vi "Update Configuration.vi"(8 "error in (no error)":errorcluster, 10 "FP Configuration":T1, 11 "Control In":refnum<class "Control.lvclass">) -> (0 "error out":errorcluster, 3 "Control In":refnum<class "Control.lvclass">)   [LabVIEW 2015, in "Front Panel Publisher.lvlib" / "Control.lvclass"]
uses:
  Control.lvclass
  Web Front Panel_class/Controls/FP Object Configuration.ctl
  Object_class/Object.lvclass
  Front Panel Publisher.lvlib
  Web Front Panel_class/Web Front Panel.lvclass
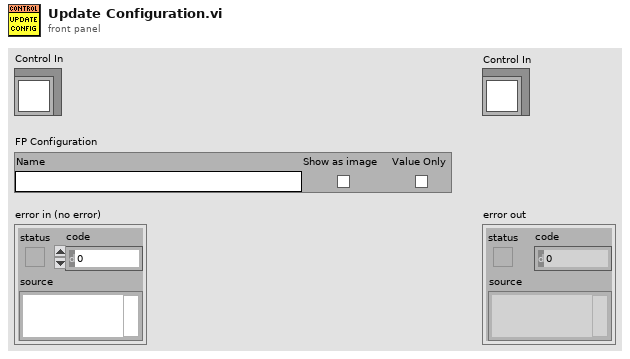
[diagram p1: front panel]
types:
  T1 = typedef "Front Panel Publisher.lvlib/Web Front Panel.lvclass/FP Object Configuration.ctl" = cluster{"Name":string, "Show as image":bool, "Value Only":bool}
  T2 = typedef "Front Panel Publisher.lvlib/Control.lvclass/Attributes.ctl" = cluster{"Description":string, "Indicator":bool, "Default Value":variant, "Control Index":i32, "Label":refnum<class "Text.lvclass">, "Caption":refnum<class "Text.lvclass">, "Image b64":string, "Use Picture":bool, "Value Only":bool}
  T3 = typedef "Front Panel Publisher.lvlib/Object.lvclass/Attributes.ctl" = cluster{"UID":i32, "Type":string, "Coordinates":T4, "Reference":refnum<vi>}
  T4 = typedef "Front Panel Publisher.lvlib/Object.lvclass/Coordinates.ctl" = cluster{"Left":i32, "Top":i32, "Height":u32, "Width":u32}
  T5 = typedef "LVRectTypeDef.ctl" = cluster{"Left":i16, "Top":i16, "Right":i16, "Bottom":i16}
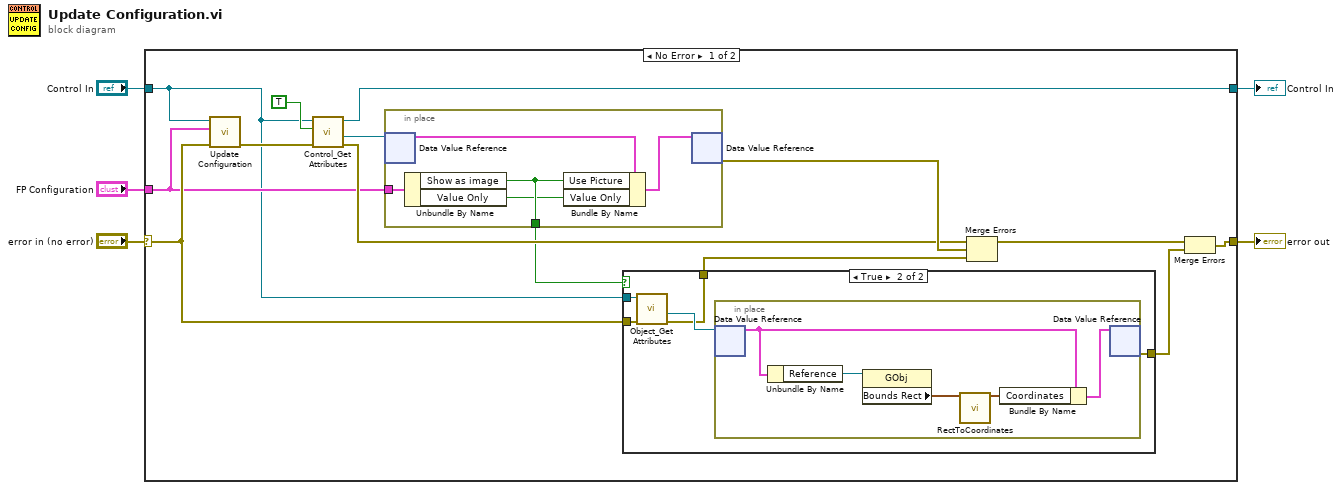
[diagram p0: block diagram]
diagram:
  n1 = case shown="No Error" "error in (no error)" {
    selector: "error in (no error)" -> [w8 w37]
    tunnel: [w10 w37] -> w4
    tunnel: [w18 w36] -> w2
    tunnel: "Control In" -> [w6 w36]
    tunnel: "FP Configuration" -> [w7 _]
    frame No Error {
      n2 = call-parent "Update Configuration.vi"("error in (no error)"=w8, "FP Configuration"=w7, "reference in"=w6) -> ("error out"=w9:errorcluster)  [unwired: 7 in, 1 out]
      n3 = call "Control_Get Attributes.vi"("error in (no error)"=w9, "Only Get DVR"=TRUE ("OnlyGetDvrReference(False)"), "Control In"=w6) -> ("error out"=w15:errorcluster, "DataRef"=w17:refnum<data-value>, "Control Out"=w18:refnum<class "Control.lvclass">)  [unwired: 5 in, 1 out]
      n4 = in-place {
        in-place-border: w7 -> [w33]
        in-place-border: [w32] -> w14
        n5 = in-place-dvr #1(w17) -> (w34:T2)  [unwired: 1 out]
        n6 = Unbundle By Name(w33) -> ("Show as image"=w32:bool, "Value Only"=w31:bool)
        n7 = Bundle By Name(cluster=w34, "Use Picture"=w32, "Value Only"=w31) -> (w35:T2)
        n8 = in-place-dvr #1(w35) -> (w19:errorcluster)  [unwired: 1 out]
      }
      n9 = case shown="True" w14 {
        tunnel: w6 -> [_ w24]
        tunnel: w8 -> [w20 w23]
        tunnel: [w20 w22] -> w13
        tunnel: [w20 w21] -> w12
        frame False {
        }
        frame True {
          n10 = call "Object_Get Attributes.vi"("error in (no error)"=w23, "Object In"=w24) -> ("error out"=w22:errorcluster, "DataRef"=w25:refnum<data-value>)  [unwired: 6 in, 2 out]
          n11 = in-place {
            n12 = in-place-dvr #2(w25) -> (w27:T3)  [unwired: 1 out]
            n13 = Unbundle By Name(w27) -> ("Reference"=w28:refnum<vi>)
            n14 = property class="GObj"(reference=w28) -> ("Bounds Rect"=w30:T5)  [unwired: 1 in, 2 out]
            n15 = call "RectToCoordinates.vi"("Rect"=w30) -> ("Coordinates"=w29:T4)  [unwired: 14 in]
            n16 = Bundle By Name(cluster=w27, "Coordinates"=w29) -> (w26:T3)
            n17 = in-place-dvr #2(w26) -> (w21:errorcluster)  [unwired: 1 out]
          }
        }
      }
      n18 = Merge Errors(w15, w19, w13) -> (w11:errorcluster)
      n19 = Merge Errors(w11, w12) -> (w10:errorcluster)
    }
    frame Error {
    }
  }
  "error out" <- w4
  "Control In" <- w2
